vi "WriteDVRTracepoint.vi"(7 "Qbus":refnum<class "Qbus.lvclass">, 8 "Replaced DVR":u32, 9 "DVR":u32, 10 "Location":u32) -> ()   [LabVIEW 2017]
uses:
  <vilib>/addons/Qbus/Qbus.lvclass
  <vilib>/addons/TraceLogger/TraceLogger.lvlib
  <vilib>/addons/InsightCM/Devices/Shared/Common/DataAccumulator/DataAccumulator.lvlib
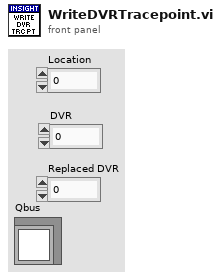
[diagram p1: front panel]
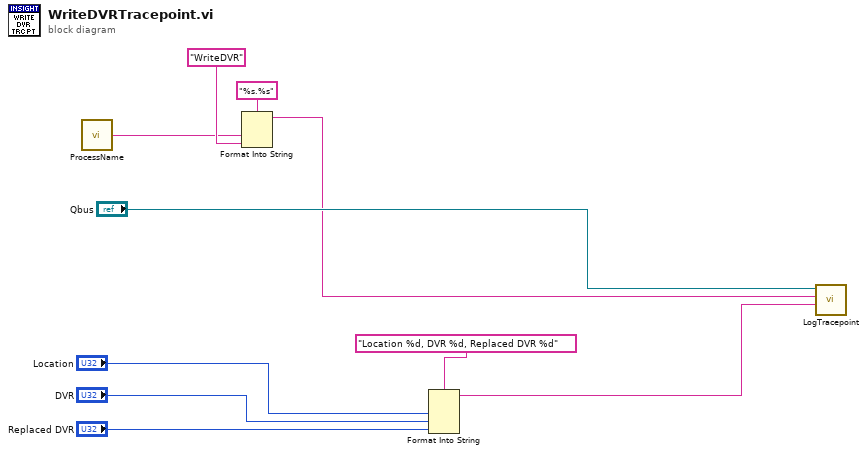
[diagram p0: block diagram]
diagram:
  n1 = call <vilib>:"ProcessName.vi"() -> ("process name"=w1:string)  [unwired: 5 in]
  n2 = Format Into String(format string="%s.%s", w1, "WriteDVR" ("tracepoint")) -> (resulting string=w6:string)  [unwired: 2 in, 1 out]
  n3 = Format Into String(format string="Location %d, DVR %d, Replaced DVR %d", "Location", "DVR", "Replaced DVR") -> (resulting string=w2:string)  [unwired: 2 in, 1 out]
  n4 = call <vilib>:"LogTracepoint.vi"("log string"=w2, "tracepoint"=w6, "qbus in"="Qbus") -> ()  [unwired: 7 in, 2 out]
